vi "PC.vi"() -> ()   [LabVIEW 2025]
uses:
  Cluster.ctl
  Enum.ctl
  <resource>/objmgr/ni.dex.rc
panel:
  out "Temperatura":i32[](graph)
  out "Puls":i32[](graph)
  out "Is Connected?":bool
  in  "IP":string
  in  "Variables":T1
  in  "stop":bool
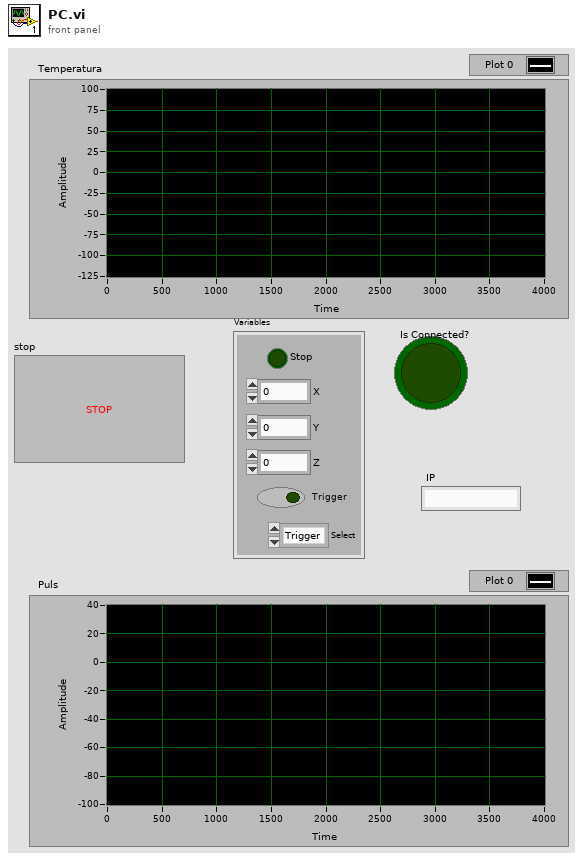
[diagram p1: front panel]
types:
  T1 = typedef "Cluster.ctl" = cluster{"X":u32, "Stop":bool, "Y":u32, "Z":u32, "Trigger":bool, "Select":T2}
  T2 = typedef "Enum.ctl" = enum16{"Trigger", "Stop", "Z", "Y", "X"}
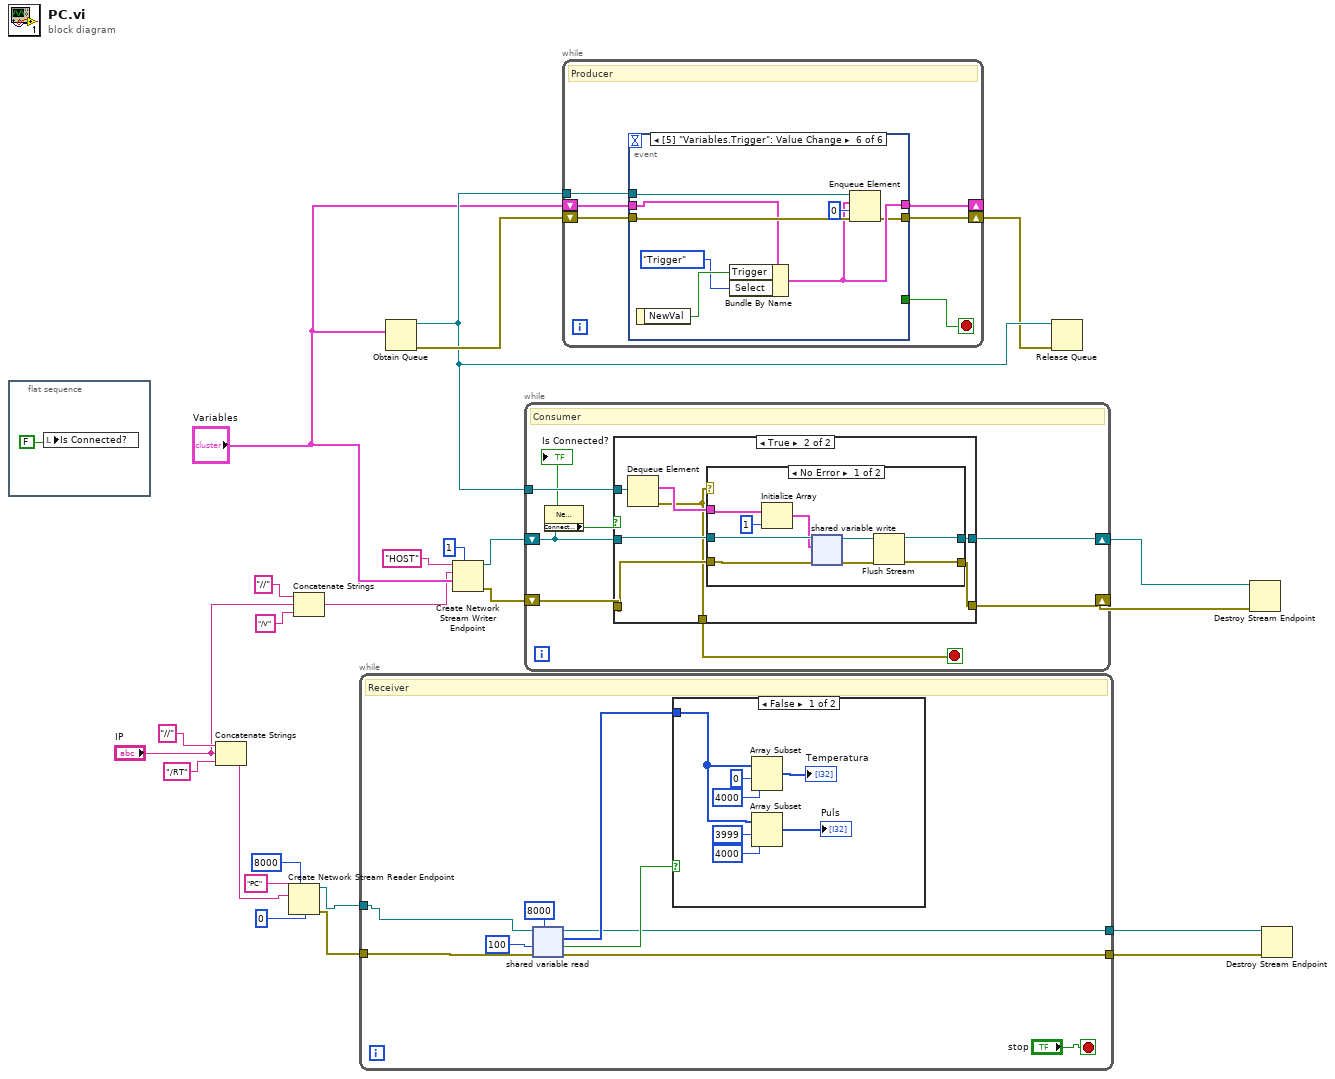
[diagram p0: block diagram]
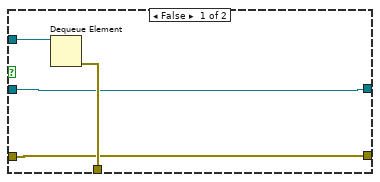
[diagram p2: hidden frame]
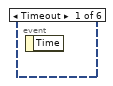
[diagram p4: hidden frame]
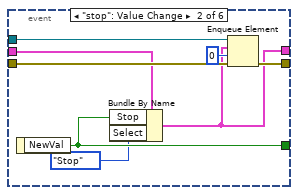
[diagram p5: hidden frame]
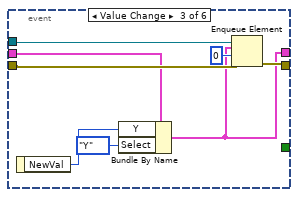
[diagram p6: hidden frame]
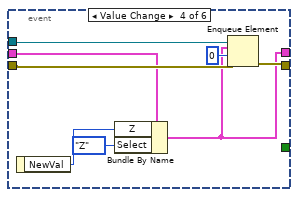
[diagram p7: hidden frame]
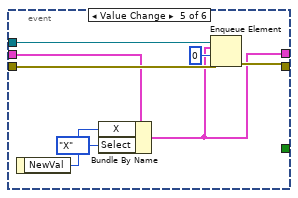
[diagram p8: hidden frame]
diagram:
  n1 = flat-sequence {
    frame #0 {
      n2 = local write "Is Connected?"(FALSE ("Is Connected")) -> ()
    }
  }
  n3 = Concatenate Strings("//" ("string"), "IP", "/RT" ("string")) -> (w4:string)
  n4 = Create Network Stream Reader Endpoint(7:8000 ("reader buffer size"), 9:0, 10:w4, 11:"PC" ("reader name")) -> (0:w3:errorcluster, 3:w6:refnum<k21>)  [unwired: 3 in]
  n5 = Concatenate Strings("//" ("string"), "IP", "/V" ("string")) -> (w9:string)
  n6 = while {
    tunnel: w6 -> [w33]
    tunnel: [w32] -> w5
    tunnel: w3 -> [w27]
    tunnel: [w26] -> w2
    stop <- "stop" stop-if-true
    # "Receiver"
    n7 = shared-variable-read(w33, w27, 100 ("timeout ms (-1)"), 8000 ("# elements")) -> (w26:refnum<k21>, w32:errorcluster, w28:bool, w30:i32[])
    n8 = case shown="False" w28 {
      tunnel: w30 -> [w37 _]
      frame False {
        n9 = Array Subset(array=w37, index=0, length=4000) -> (→"Temperatura":i32[])
        n10 = Array Subset(array=w37, index=3999, length=4000) -> (→"Puls":i32[])
      }
      frame True {
      }
    }
  }
  n11 = Obtain Queue(element data type="Variables") -> (queue out=w23:refnum<queue>, error out=w24:errorcluster)  [unwired: 4 in, 1 out]
  n12 = Create Network Stream Writer Endpoint(7:1 ("writer buffer size"), 9:"Variables", 10:w9, 11:"HOST" ("writer name")) -> (0:w7:errorcluster, 3:w8:refnum<k21>)  [unwired: 3 in]
  n13 = while {
    tunnel: w23 -> [w45]
    shift-right: [w42] -> w1
    shift-left: w8 -> [w44]
    shift-right: [w47] -> w22
    shift-left: w7 -> [w48]
    stop <- w46 stop-if-true
    # "Consumer"
    n14 = property class="Network Stream Endpoint"(reference=w44) -> ("Connected"=w43:bool)  [unwired: 1 in, 2 out]
    "Is Connected?" <- w43
    n15 = case shown="True" w43 {
      tunnel: w45 -> [w51 w59]
      tunnel: w48 -> [w49 w57]
      tunnel: w44 -> [w50 w56]
      tunnel: [w50 w55] -> w42
      tunnel: [w49 w54] -> w47
      tunnel: [w52 w53] -> w46
      frame False {
        n16 = Dequeue Element(queue=w51) -> (error out=w52:errorcluster)  [unwired: 2 in, 3 out]
      }
      frame True {
        n17 = Dequeue Element(queue=w59) -> (element=w58:T1, error out=w53:errorcluster)  [unwired: 2 in, 2 out]
        n18 = case shown="No Error" w53 {
          tunnel: w58 -> [w68 _]
          tunnel: w57 -> [w66 _]
          tunnel: w56 -> [w65 _]
          tunnel: [w62 _] -> w55
          tunnel: [w60 _] -> w54
          frame No Error {
            n19 = Initialize Array(w68, 1 ("dimension size")) -> (w64:T1[])
            n20 = shared-variable-write(w65, w66, w64) -> (w63:refnum<k21>, w61:errorcluster)  [unwired: 1 in, 1 out]
            n21 = Flush Stream(8:w61, 11:w63) -> (0:w60:errorcluster, 3:w62:refnum<k21>)  [unwired: 2 in, 1 out]
          }
          frame Error {
          }
        }
      }
    }
  }
  n22 = while {
    tunnel: w23 -> [w74]
    shift-right: [w72] -> w21
    shift-left: w24 -> [w73]
    shift-right: [w70] -> _
    shift-left: "Variables" -> [w71]
    stop <- w69 stop-if-true
    # "Producer"
    n23 = event shown="[5] \"Variables.Trigger\": Value Change" {
      selector: _ -> [_ _ _ _ _ _]
      dyn-events: _ -> [_ _ _ _ _ _]
      timeout: _ -> [_ _ _ _ _ _]
      tunnel: w74 -> [_ w82 w89 w96 w106 w113]
      tunnel: w73 -> [_ w80 w88 w95 w105 w112]
      tunnel: [_ w81 w85 w97 w104 w109] -> w72
      tunnel: w71 -> [_ w78 w87 w94 w102 w111]
      tunnel: [_ w77 w84 w92 w100 w110] -> w70
      tunnel: [_ w76 _ _ _ _] -> w69
      event Timeout {
        n24 = event-data() -> ()  [unwired: 1 in, 1 out]
      }
      event "stop": Value Change {
        n25 = event-data() -> ("NewVal"=w76:bool)  [unwired: 1 in]
        n26 = Bundle By Name(cluster=w78, "Stop"=w76, "Select"=Enum."Stop") -> (w77:T1)
        n27 = Enqueue Element(queue=w82, element=w77, timeout in ms (-1)=0, error in (no error)=w80) -> (error out=w81:errorcluster)  [unwired: 2 out]
      }
      event Value Change {
        n28 = event-data() -> ("NewVal"=w86:u32)  [unwired: 1 in]
        n29 = Bundle By Name(cluster=w87, "Y"=w86, "Select"=Enum."Y") -> (w84:T1)
        n30 = Enqueue Element(queue=w89, element=w84, timeout in ms (-1)=0, error in (no error)=w88) -> (error out=w85:errorcluster)  [unwired: 2 out]
      }
      event Value Change {
        n31 = event-data() -> ("NewVal"=w93:u32)  [unwired: 1 in]
        n32 = Bundle By Name(cluster=w94, "Z"=w93, "Select"=Enum."Z") -> (w92:T1)
        n33 = Enqueue Element(queue=w96, element=w92, timeout in ms (-1)=0, error in (no error)=w95) -> (error out=w97:errorcluster)  [unwired: 2 out]
      }
      event Value Change {
        n34 = event-data() -> ("NewVal"=w101:u32)  [unwired: 1 in]
        n35 = Bundle By Name(cluster=w102, "X"=w101, "Select"=Enum."X") -> (w100:T1)
        n36 = Enqueue Element(queue=w106, element=w100, timeout in ms (-1)=0, error in (no error)=w105) -> (error out=w104:errorcluster)  [unwired: 2 out]
      }
      event Value Change {
        n37 = event-data() -> ("NewVal"=w108:bool)  [unwired: 1 in]
        n38 = Bundle By Name(cluster=w111, "Trigger"=w108, "Select"=Enum."Trigger") -> (w110:T1)
        n39 = Enqueue Element(queue=w113, element=w110, timeout in ms (-1)=0, error in (no error)=w112) -> (error out=w109:errorcluster)  [unwired: 2 out]
      }
    }
  }
  n40 = Release Queue(queue=w23, error in (no error)=w21) -> ()  [unwired: 1 in, 3 out]
  n41 = Destroy Stream Endpoint(8:w22, 11:w1) -> ()  [unwired: 1 out]
  n42 = Destroy Stream Endpoint(8:w5, 11:w2) -> ()  [unwired: 1 out]
